vi "Lab Panel V5.10.vi"() -> ()   [LabVIEW 2013] (continued)
                          tunnel: w3985 -> [_ w4027]
                          tunnel: w3984 -> [_ w4019]
                          frame False {
                          }
                          frame True {
                            n2197 = local read "TDMS LAB02-1"() -> (w4032:refnum<k34>)
                            n2198 = Build Array(w4029) -> (w4024:dbl[])
                            n2199 = Build Array(w4027) -> (w4023:dbl[])
                            n2200 = Build Array(w4034) -> (w4022:dbl[])
                            n2201 = Build Array(w4035) -> (w4021:dbl[])
                            n2202 = Build Array(w4030) -> (w4026:dbl[])
                            n2203 = Build Array(w4028) -> (w4025:dbl[])
                            n2204 = Build Array(w4033) -> (w4020:dbl[])
                            n2205 = Build Array("AMPS ON", "AMPS OFF", "VOLTS", "PF", "TEMP Live", "TEMP Neut", "CYCLE") -> (w4003:string[])
                            n2206 = Bundle By Name("Y"=w4026, "t0"=w4019) -> (w4018:waveform(dbl))  [unwired: 1 in]
                            n2207 = Bundle By Name("Y"=w4025, "t0"=w4019) -> (w4017:waveform(dbl))  [unwired: 1 in]
                            n2208 = Bundle By Name("Y"=w4024, "t0"=w4019) -> (w4016:waveform(dbl))  [unwired: 1 in]
                            n2209 = Bundle By Name("Y"=w4023, "t0"=w4019) -> (w4015:waveform(dbl))  [unwired: 1 in]
                            n2210 = Bundle By Name("Y"=w4022, "t0"=w4019) -> (w4014:waveform(dbl))  [unwired: 1 in]
                            n2211 = Bundle By Name("Y"=w4021, "t0"=w4019) -> (w4013:waveform(dbl))  [unwired: 1 in]
                            n2212 = Bundle By Name("Y"=w4020, "t0"=w4019) -> (w4012:waveform(dbl))  [unwired: 1 in]
                            n2213 = Build Array(w4018, w4017, w4016, w4015, w4014, w4013, w4012) -> (w4011:waveform(dbl)[])
                            n2214 = TDMS Write(0:w4032, 5:"TEST VALUES", 7:w4003, 9:w4011) -> (4:w4002:refnum<k34>, 6:w4001:string, 15:w4000:errorcluster)  [unwired: 2 in, 1 out]
                            n2215 = TDMS Write(0:w4002, 5:w4001, 7:"TIME", 9:w3998, 11:w4000) -> (15:w3997:errorcluster)  [unwired: 1 in, 3 out]
                            n2216 = local write "data file error"(w3997) -> ()
                          }
                        }
                      }
                    }
                  }
                }
              }
              frame #3 {
                n2217 = case shown="True" w4036 {
                  tunnel: w4040 -> [_ w4045]
                  tunnel: w4039 -> [_ w4044]
                  tunnel: w4038 -> [_ w4042]
                  tunnel: w4037 -> [_ w4041]
                  frame False {
                  }
                  frame True {
                    n2218 = local read "DISP LAB02-2"() -> (w4046:T4)
                    n2219 = local read "SIG LAB02-2"() -> (w4047:T2)
                    n2220 = local read "ON L02-2"() -> (w4043:cluster{"amps":dbl, "volts":dbl, "pf":dbl})
                    n2221 = Unbundle(w4047) -> ("AMPS"=w4053:dbl, "VOLTS"=w4051:dbl, "PF"=w4050:dbl, "Tmp Live"=w4049:dbl, "Tmp Neut"=w4052:dbl)
                    n2222 = Unbundle(w4046) -> ("CYCLE"=w4048:dbl)  [unwired: 2 out]
                    n2223 = stacked-sequence {
                      tunnel: w4053 -> [w4057 w4076]
                      tunnel: w4052 -> [_ w4075]
                      tunnel: w4051 -> [w4056 w4074]
                      tunnel: w4050 -> [w4055 w4073]
                      tunnel: w4049 -> [_ w4072]
                      tunnel: w4048 -> [_ w4071]
                      tunnel: w4045 -> [_ w4070]
                      tunnel: w4044 -> [w4058 _]
                      tunnel: w4043 -> [w4054 w4068]
                      tunnel: w4042 -> [_ w4069]
                      tunnel: w4041 -> [_ w4064]
                      frame #0 {
                        n2224 = case shown="True" w4058 {
                          tunnel: w4057 -> [_ w4063]
                          tunnel: w4056 -> [_ w4062]
                          tunnel: w4055 -> [_ w4061]
                          tunnel: w4054 -> [_ w4059]
                          frame False {
                          }
                          frame True {
                            n2225 = Bundle(cluster=w4059, "amps"=w4063, "volts"=w4062, "pf"=w4061) -> (w4060:cluster{"amps":dbl, "volts":dbl, "pf":dbl})
                            n2226 = local write "ON L02-2"(w4060) -> ()
                          }
                        }
                      }
                      frame #1 {
                        n2227 = Unbundle(w4068) -> ("amps"=w4067:dbl, "volts"=w4066:dbl, "pf"=w4065:dbl)
                        n2228 = case shown="True" w4069 {
                          tunnel: w4076 -> [_ w4108]
                          tunnel: w4075 -> [_ w4115]
                          tunnel: w4074 -> [_ _]
                          tunnel: w4073 -> [_ _]
                          tunnel: w4072 -> [_ w4114]
                          tunnel: w4071 -> [_ w4113]
                          tunnel: w4070 -> [_ w4078]
                          tunnel: w4067 -> [_ w4110]
                          tunnel: w4066 -> [_ w4109]
                          tunnel: w4065 -> [_ w4107]
                          tunnel: w4064 -> [_ w4099]
                          frame False {
                          }
                          frame True {
                            n2229 = local read "TDMS LAB02-2"() -> (w4112:refnum<k34>)
                            n2230 = Build Array(w4109) -> (w4104:dbl[])
                            n2231 = Build Array(w4107) -> (w4103:dbl[])
                            n2232 = Build Array(w4114) -> (w4102:dbl[])
                            n2233 = Build Array(w4115) -> (w4101:dbl[])
                            n2234 = Build Array(w4110) -> (w4106:dbl[])
                            n2235 = Build Array(w4108) -> (w4105:dbl[])
                            n2236 = Build Array(w4113) -> (w4100:dbl[])
                            n2237 = Build Array("AMPS ON", "AMPS OFF", "VOLTS", "PF", "TEMP Live", "TEMP Neut", "CYCLE") -> (w4083:string[])
                            n2238 = Bundle By Name("Y"=w4106, "t0"=w4099) -> (w4098:waveform(dbl))  [unwired: 1 in]
                            n2239 = Bundle By Name("Y"=w4105, "t0"=w4099) -> (w4097:waveform(dbl))  [unwired: 1 in]
                            n2240 = Bundle By Name("Y"=w4104, "t0"=w4099) -> (w4096:waveform(dbl))  [unwired: 1 in]
                            n2241 = Bundle By Name("Y"=w4103, "t0"=w4099) -> (w4095:waveform(dbl))  [unwired: 1 in]
                            n2242 = Bundle By Name("Y"=w4102, "t0"=w4099) -> (w4094:waveform(dbl))  [unwired: 1 in]
                            n2243 = Bundle By Name("Y"=w4101, "t0"=w4099) -> (w4093:waveform(dbl))  [unwired: 1 in]
                            n2244 = Bundle By Name("Y"=w4100, "t0"=w4099) -> (w4092:waveform(dbl))  [unwired: 1 in]
                            n2245 = Build Array(w4098, w4097, w4096, w4095, w4094, w4093, w4092) -> (w4091:waveform(dbl)[])
                            n2246 = TDMS Write(0:w4112, 5:"TEST VALUES", 7:w4083, 9:w4091) -> (4:w4082:refnum<k34>, 6:w4081:string, 15:w4080:errorcluster)  [unwired: 2 in, 1 out]
                            n2247 = TDMS Write(0:w4082, 5:w4081, 7:"TIME", 9:w4078, 11:w4080) -> (15:w4077:errorcluster)  [unwired: 1 in, 3 out]
                            n2248 = local write "data file error"(w4077) -> ()
                          }
                        }
                      }
                    }
                  }
                }
              }
              frame #4 {
                n2249 = case shown="True" w4116 {
                  tunnel: w4120 -> [_ w4125]
                  tunnel: w4119 -> [_ w4124]
                  tunnel: w4118 -> [_ w4122]
                  tunnel: w4117 -> [_ w4121]
                  frame False {
                  }
                  frame True {
                    n2250 = local read "DISP LAB03-1"() -> (w4126:T4)
                    n2251 = local read "SIG LAB03-1"() -> (w4127:T2)
                    n2252 = local read "ON L03-1"() -> (w4123:cluster{"amps":dbl, "volts":dbl, "pf":dbl})
                    n2253 = Unbundle(w4127) -> ("AMPS"=w4133:dbl, "VOLTS"=w4131:dbl, "PF"=w4130:dbl, "Tmp Live"=w4129:dbl, "Tmp Neut"=w4132:dbl)
                    n2254 = Unbundle(w4126) -> ("CYCLE"=w4128:dbl)  [unwired: 2 out]
                    n2255 = stacked-sequence {
                      tunnel: w4133 -> [w4137 w4156]
                      tunnel: w4132 -> [_ w4155]
                      tunnel: w4131 -> [w4136 w4154]
                      tunnel: w4130 -> [w4135 w4153]
                      tunnel: w4129 -> [_ w4152]
                      tunnel: w4128 -> [_ w4151]
                      tunnel: w4125 -> [_ w4150]
                      tunnel: w4124 -> [w4138 _]
                      tunnel: w4123 -> [w4134 w4148]
                      tunnel: w4122 -> [_ w4149]
                      tunnel: w4121 -> [_ w4144]
                      frame #0 {
                        n2256 = case shown="True" w4138 {
                          tunnel: w4137 -> [_ w4143]
                          tunnel: w4136 -> [_ w4142]
                          tunnel: w4135 -> [_ w4141]
                          tunnel: w4134 -> [_ w4139]
                          frame False {
                          }
                          frame True {
                            n2257 = Bundle(cluster=w4139, "amps"=w4143, "volts"=w4142, "pf"=w4141) -> (w4140:cluster{"amps":dbl, "volts":dbl, "pf":dbl})
                            n2258 = local write "ON L03-1"(w4140) -> ()
                          }
                        }
                      }
                      frame #1 {
                        n2259 = Unbundle(w4148) -> ("amps"=w4147:dbl, "volts"=w4146:dbl, "pf"=w4145:dbl)
                        n2260 = case shown="True" w4149 {
                          tunnel: w4156 -> [_ w4188]
                          tunnel: w4155 -> [_ w4195]
                          tunnel: w4154 -> [_ _]
                          tunnel: w4153 -> [_ _]
                          tunnel: w4152 -> [_ w4194]
                          tunnel: w4151 -> [_ w4193]
                          tunnel: w4150 -> [_ w4158]
                          tunnel: w4147 -> [_ w4190]
                          tunnel: w4146 -> [_ w4189]
                          tunnel: w4145 -> [_ w4187]
                          tunnel: w4144 -> [_ w4179]
                          frame False {
                          }
                          frame True {
                            n2261 = local read "TDMS LAB03-1"() -> (w4192:refnum<k34>)
                            n2262 = Build Array(w4189) -> (w4184:dbl[])
                            n2263 = Build Array(w4187) -> (w4183:dbl[])
                            n2264 = Build Array(w4194) -> (w4182:dbl[])
                            n2265 = Build Array(w4195) -> (w4181:dbl[])
                            n2266 = Build Array(w4190) -> (w4186:dbl[])
                            n2267 = Build Array(w4188) -> (w4185:dbl[])
                            n2268 = Build Array(w4193) -> (w4180:dbl[])
                            n2269 = Build Array("AMPS ON", "AMPS OFF", "VOLTS", "PF", "TEMP Live", "TEMP Neut", "CYCLE") -> (w4163:string[])
                            n2270 = Bundle By Name("Y"=w4186, "t0"=w4179) -> (w4178:waveform(dbl))  [unwired: 1 in]
                            n2271 = Bundle By Name("Y"=w4185, "t0"=w4179) -> (w4177:waveform(dbl))  [unwired: 1 in]
                            n2272 = Bundle By Name("Y"=w4184, "t0"=w4179) -> (w4176:waveform(dbl))  [unwired: 1 in]
                            n2273 = Bundle By Name("Y"=w4183, "t0"=w4179) -> (w4175:waveform(dbl))  [unwired: 1 in]
                            n2274 = Bundle By Name("Y"=w4182, "t0"=w4179) -> (w4174:waveform(dbl))  [unwired: 1 in]
                            n2275 = Bundle By Name("Y"=w4181, "t0"=w4179) -> (w4173:waveform(dbl))  [unwired: 1 in]
                            n2276 = Bundle By Name("Y"=w4180, "t0"=w4179) -> (w4172:waveform(dbl))  [unwired: 1 in]
                            n2277 = Build Array(w4178, w4177, w4176, w4175, w4174, w4173, w4172) -> (w4171:waveform(dbl)[])
                            n2278 = TDMS Write(0:w4192, 5:"TEST VALUES", 7:w4163, 9:w4171) -> (4:w4162:refnum<k34>, 6:w4161:string, 15:w4160:errorcluster)  [unwired: 2 in, 1 out]
                            n2279 = TDMS Write(0:w4162, 5:w4161, 7:"TIME", 9:w4158, 11:w4160) -> (15:w4157:errorcluster)  [unwired: 1 in, 3 out]
                            n2280 = local write "data file error"(w4157) -> ()
                          }
                        }
                      }
                    }
                  }
                }
              }
              frame #5 {
                n2281 = case shown="True" w4196 {
                  tunnel: w4200 -> [_ w4205]
                  tunnel: w4199 -> [_ w4204]
                  tunnel: w4198 -> [_ w4202]
                  tunnel: w4197 -> [_ w4201]
                  frame False {
                  }
                  frame True {
                    n2282 = local read "DISP LAB03-2"() -> (w4206:T4)
                    n2283 = local read "SIG LAB03-2"() -> (w4207:T2)
                    n2284 = local read "ON L03-2"() -> (w4203:cluster{"amps":dbl, "volts":dbl, "pf":dbl})
                    n2285 = Unbundle(w4207) -> ("AMPS"=w4213:dbl, "VOLTS"=w4211:dbl, "PF"=w4210:dbl, "Tmp Live"=w4209:dbl, "Tmp Neut"=w4212:dbl)
                    n2286 = Unbundle(w4206) -> ("CYCLE"=w4208:dbl)  [unwired: 2 out]
                    n2287 = stacked-sequence {
                      tunnel: w4213 -> [w4217 w4236]
                      tunnel: w4212 -> [_ w4235]
                      tunnel: w4211 -> [w4216 w4234]
                      tunnel: w4210 -> [w4215 w4233]
                      tunnel: w4209 -> [_ w4232]
                      tunnel: w4208 -> [_ w4231]
                      tunnel: w4205 -> [_ w4230]
                      tunnel: w4204 -> [w4218 _]
                      tunnel: w4203 -> [w4214 w4228]
                      tunnel: w4202 -> [_ w4229]
                      tunnel: w4201 -> [_ w4224]
                      frame #0 {
                        n2288 = case shown="True" w4218 {
                          tunnel: w4217 -> [_ w4223]
                          tunnel: w4216 -> [_ w4222]
                          tunnel: w4215 -> [_ w4221]
                          tunnel: w4214 -> [_ w4219]
                          frame False {
                          }
                          frame True {
                            n2289 = Bundle(cluster=w4219, "amps"=w4223, "volts"=w4222, "pf"=w4221) -> (w4220:cluster{"amps":dbl, "volts":dbl, "pf":dbl})
                            n2290 = local write "ON L03-2"(w4220) -> ()
                          }
                        }
                      }
                      frame #1 {
                        n2291 = Unbundle(w4228) -> ("amps"=w4227:dbl, "volts"=w4226:dbl, "pf"=w4225:dbl)
                        n2292 = case shown="True" w4229 {
                          tunnel: w4236 -> [_ w4268]
                          tunnel: w4235 -> [_ w4275]
                          tunnel: w4234 -> [_ _]
                          tunnel: w4233 -> [_ _]
                          tunnel: w4232 -> [_ w4274]
                          tunnel: w4231 -> [_ w4273]
                          tunnel: w4230 -> [_ w4238]
                          tunnel: w4227 -> [_ w4270]
                          tunnel: w4226 -> [_ w4269]
                          tunnel: w4225 -> [_ w4267]
                          tunnel: w4224 -> [_ w4259]
                          frame False {
                          }
                          frame True {
                            n2293 = local read "TDMS LAB03-2"() -> (w4272:refnum<k34>)
                            n2294 = Build Array(w4269) -> (w4264:dbl[])
                            n2295 = Build Array(w4267) -> (w4263:dbl[])
                            n2296 = Build Array(w4274) -> (w4262:dbl[])
                            n2297 = Build Array(w4275) -> (w4261:dbl[])
                            n2298 = Build Array(w4270) -> (w4266:dbl[])
                            n2299 = Build Array(w4268) -> (w4265:dbl[])
                            n2300 = Build Array(w4273) -> (w4260:dbl[])
                            n2301 = Build Array("AMPS ON", "AMPS OFF", "VOLTS", "PF", "TEMP Live", "TEMP Neut", "CYCLE") -> (w4243:string[])
                            n2302 = Bundle By Name("Y"=w4266, "t0"=w4259) -> (w4258:waveform(dbl))  [unwired: 1 in]
                            n2303 = Bundle By Name("Y"=w4265, "t0"=w4259) -> (w4257:waveform(dbl))  [unwired: 1 in]
                            n2304 = Bundle By Name("Y"=w4264, "t0"=w4259) -> (w4256:waveform(dbl))  [unwired: 1 in]
                            n2305 = Bundle By Name("Y"=w4263, "t0"=w4259) -> (w4255:waveform(dbl))  [unwired: 1 in]
                            n2306 = Bundle By Name("Y"=w4262, "t0"=w4259) -> (w4254:waveform(dbl))  [unwired: 1 in]
                            n2307 = Bundle By Name("Y"=w4261, "t0"=w4259) -> (w4253:waveform(dbl))  [unwired: 1 in]
                            n2308 = Bundle By Name("Y"=w4260, "t0"=w4259) -> (w4252:waveform(dbl))  [unwired: 1 in]
                            n2309 = Build Array(w4258, w4257, w4256, w4255, w4254, w4253, w4252) -> (w4251:waveform(dbl)[])
                            n2310 = TDMS Write(0:w4272, 5:"TEST VALUES", 7:w4243, 9:w4251) -> (4:w4242:refnum<k34>, 6:w4241:string, 15:w4240:errorcluster)  [unwired: 2 in, 1 out]
                            n2311 = TDMS Write(0:w4242, 5:w4241, 7:"TIME", 9:w4238, 11:w4240) -> (15:w4237:errorcluster)  [unwired: 1 in, 3 out]
                            n2312 = local write "data file error"(w4237) -> ()
                          }
                        }
                      }
                    }
                  }
                }
              }
              frame #6 {
                n2313 = case shown="True" w4276 {
                  tunnel: w4280 -> [_ w4285]
                  tunnel: w4279 -> [_ w4284]
                  tunnel: w4278 -> [_ w4282]
                  tunnel: w4277 -> [_ w4281]
                  frame False {
                  }
                  frame True {
                    n2314 = local read "DISP LAB04-1"() -> (w4286:T4)
                    n2315 = local read "SIG LAB04-1"() -> (w4287:T2)
                    n2316 = local read "ON L04-1"() -> (w4283:cluster{"amps":dbl, "volts":dbl, "pf":dbl})
                    n2317 = Unbundle(w4287) -> ("AMPS"=w4293:dbl, "VOLTS"=w4291:dbl, "PF"=w4290:dbl, "Tmp Live"=w4289:dbl, "Tmp Neut"=w4292:dbl)
                    n2318 = Unbundle(w4286) -> ("CYCLE"=w4288:dbl)  [unwired: 2 out]
                    n2319 = stacked-sequence {
                      tunnel: w4293 -> [w4297 w4316]
                      tunnel: w4292 -> [_ w4315]
                      tunnel: w4291 -> [w4296 w4314]
                      tunnel: w4290 -> [w4295 w4313]
                      tunnel: w4289 -> [_ w4312]
                      tunnel: w4288 -> [_ w4311]
                      tunnel: w4285 -> [_ w4310]
                      tunnel: w4284 -> [w4298 _]
                      tunnel: w4283 -> [w4294 w4308]
                      tunnel: w4282 -> [_ w4309]
                      tunnel: w4281 -> [_ w4304]
                      frame #0 {
                        n2320 = case shown="True" w4298 {
                          tunnel: w4297 -> [_ w4303]
                          tunnel: w4296 -> [_ w4302]
                          tunnel: w4295 -> [_ w4301]
                          tunnel: w4294 -> [_ w4299]
                          frame False {
                          }
                          frame True {
                            n2321 = Bundle(cluster=w4299, "amps"=w4303, "volts"=w4302, "pf"=w4301) -> (w4300:cluster{"amps":dbl, "volts":dbl, "pf":dbl})
                            n2322 = local write "ON L04-1"(w4300) -> ()
                          }
                        }
                      }
                      frame #1 {
                        n2323 = Unbundle(w4308) -> ("amps"=w4307:dbl, "volts"=w4306:dbl, "pf"=w4305:dbl)
                        n2324 = case shown="True" w4309 {
                          tunnel: w4316 -> [_ w4348]
                          tunnel: w4315 -> [_ w4355]
                          tunnel: w4314 -> [_ _]
                          tunnel: w4313 -> [_ _]
                          tunnel: w4312 -> [_ w4354]
                          tunnel: w4311 -> [_ w4353]
                          tunnel: w4310 -> [_ w4318]
                          tunnel: w4307 -> [_ w4350]
                          tunnel: w4306 -> [_ w4349]
                          tunnel: w4305 -> [_ w4347]
                          tunnel: w4304 -> [_ w4339]
                          frame False {
                          }
                          frame True {
                            n2325 = local read "TDMS LAB04-1"() -> (w4352:refnum<k34>)
                            n2326 = Build Array(w4349) -> (w4344:dbl[])
                            n2327 = Build Array(w4347) -> (w4343:dbl[])
                            n2328 = Build Array(w4354) -> (w4342:dbl[])
                            n2329 = Build Array(w4355) -> (w4341:dbl[])
                            n2330 = Build Array(w4350) -> (w4346:dbl[])
                            n2331 = Build Array(w4348) -> (w4345:dbl[])
                            n2332 = Build Array(w4353) -> (w4340:dbl[])
                            n2333 = Build Array("AMPS ON", "AMPS OFF", "VOLTS", "PF", "TEMP Live", "TEMP Neut", "CYCLE") -> (w4323:string[])
                            n2334 = Bundle By Name("Y"=w4346, "t0"=w4339) -> (w4338:waveform(dbl))  [unwired: 1 in]
                            n2335 = Bundle By Name("Y"=w4345, "t0"=w4339) -> (w4337:waveform(dbl))  [unwired: 1 in]
                            n2336 = Bundle By Name("Y"=w4344, "t0"=w4339) -> (w4336:waveform(dbl))  [unwired: 1 in]
                            n2337 = Bundle By Name("Y"=w4343, "t0"=w4339) -> (w4335:waveform(dbl))  [unwired: 1 in]
                            n2338 = Bundle By Name("Y"=w4342, "t0"=w4339) -> (w4334:waveform(dbl))  [unwired: 1 in]
                            n2339 = Bundle By Name("Y"=w4341, "t0"=w4339) -> (w4333:waveform(dbl))  [unwired: 1 in]
                            n2340 = Bundle By Name("Y"=w4340, "t0"=w4339) -> (w4332:waveform(dbl))  [unwired: 1 in]
                            n2341 = Build Array(w4338, w4337, w4336, w4335, w4334, w4333, w4332) -> (w4331:waveform(dbl)[])
                            n2342 = TDMS Write(0:w4352, 5:"TEST VALUES", 7:w4323, 9:w4331) -> (4:w4322:refnum<k34>, 6:w4321:string, 15:w4320:errorcluster)  [unwired: 2 in, 1 out]
                            n2343 = TDMS Write(0:w4322, 5:w4321, 7:"TIME", 9:w4318, 11:w4320) -> (15:w4317:errorcluster)  [unwired: 1 in, 3 out]
                            n2344 = local write "data file error"(w4317) -> ()
                          }
                        }
                      }
                    }
                  }
                }
              }
              frame #7 {
                n2345 = case shown="True" w4356 {
                  tunnel: w4360 -> [_ w4365]
                  tunnel: w4359 -> [_ w4364]
                  tunnel: w4358 -> [_ w4362]
                  tunnel: w4357 -> [_ w4361]
                  frame False {
                  }
                  frame True {
                    n2346 = local read "DISP LAB04-2"() -> (w4366:T4)
                    n2347 = local read "SIG LAB04-2"() -> (w4367:T2)
                    n2348 = local read "ON L04-2"() -> (w4363:cluster{"amps":dbl, "volts":dbl, "pf":dbl})
                    n2349 = Unbundle(w4367) -> ("AMPS"=w4373:dbl, "VOLTS"=w4371:dbl, "PF"=w4370:dbl, "Tmp Live"=w4369:dbl, "Tmp Neut"=w4372:dbl)
                    n2350 = Unbundle(w4366) -> ("CYCLE"=w4368:dbl)  [unwired: 2 out]
                    n2351 = stacked-sequence {
                      tunnel: w4373 -> [w4377 w4396]
                      tunnel: w4372 -> [_ w4395]
                      tunnel: w4371 -> [w4376 w4394]
                      tunnel: w4370 -> [w4375 w4393]
                      tunnel: w4369 -> [_ w4392]
                      tunnel: w4368 -> [_ w4391]
                      tunnel: w4365 -> [_ w4390]
                      tunnel: w4364 -> [w4378 _]
                      tunnel: w4363 -> [w4374 w4388]
                      tunnel: w4362 -> [_ w4389]
                      tunnel: w4361 -> [_ w4384]
                      frame #0 {
                        n2352 = case shown="True" w4378 {
                          tunnel: w4377 -> [_ w4383]
                          tunnel: w4376 -> [_ w4382]
                          tunnel: w4375 -> [_ w4381]
                          tunnel: w4374 -> [_ w4379]
                          frame False {
                          }
                          frame True {
                            n2353 = Bundle(cluster=w4379, "amps"=w4383, "volts"=w4382, "pf"=w4381) -> (w4380:cluster{"amps":dbl, "volts":dbl, "pf":dbl})
                            n2354 = local write "ON L04-2"(w4380) -> ()
                          }
                        }
                      }
                      frame #1 {
                        n2355 = Unbundle(w4388) -> ("amps"=w4387:dbl, "volts"=w4386:dbl, "pf"=w4385:dbl)
                        n2356 = case shown="True" w4389 {
                          tunnel: w4396 -> [_ w4428]
                          tunnel: w4395 -> [_ w4435]
                          tunnel: w4394 -> [_ _]
                          tunnel: w4393 -> [_ _]
                          tunnel: w4392 -> [_ w4434]
                          tunnel: w4391 -> [_ w4433]
                          tunnel: w4390 -> [_ w4398]
                          tunnel: w4387 -> [_ w4430]
                          tunnel: w4386 -> [_ w4429]
                          tunnel: w4385 -> [_ w4427]
                          tunnel: w4384 -> [_ w4419]
                          frame False {
                          }
                          frame True {
                            n2357 = local read "TDMS LAB04-2"() -> (w4432:refnum<k34>)
                            n2358 = Build Array(w4429) -> (w4424:dbl[])
                            n2359 = Build Array(w4427) -> (w4423:dbl[])
                            n2360 = Build Array(w4434) -> (w4422:dbl[])
                            n2361 = Build Array(w4435) -> (w4421:dbl[])
                            n2362 = Build Array(w4430) -> (w4426:dbl[])
                            n2363 = Build Array(w4428) -> (w4425:dbl[])
                            n2364 = Build Array(w4433) -> (w4420:dbl[])
                            n2365 = Build Array("AMPS ON", "AMPS OFF", "VOLTS", "PF", "TEMP Live", "TEMP Neut", "CYCLE") -> (w4403:string[])
                            n2366 = Bundle By Name("Y"=w4426, "t0"=w4419) -> (w4418:waveform(dbl))  [unwired: 1 in]
                            n2367 = Bundle By Name("Y"=w4425, "t0"=w4419) -> (w4417:waveform(dbl))  [unwired: 1 in]
                            n2368 = Bundle By Name("Y"=w4424, "t0"=w4419) -> (w4416:waveform(dbl))  [unwired: 1 in]
                            n2369 = Bundle By Name("Y"=w4423, "t0"=w4419) -> (w4415:waveform(dbl))  [unwired: 1 in]
                            n2370 = Bundle By Name("Y"=w4422, "t0"=w4419) -> (w4414:waveform(dbl))  [unwired: 1 in]
                            n2371 = Bundle By Name("Y"=w4421, "t0"=w4419) -> (w4413:waveform(dbl))  [unwired: 1 in]
                            n2372 = Bundle By Name("Y"=w4420, "t0"=w4419) -> (w4412:waveform(dbl))  [unwired: 1 in]
                            n2373 = Build Array(w4418, w4417, w4416, w4415, w4414, w4413, w4412) -> (w4411:waveform(dbl)[])
                            n2374 = TDMS Write(0:w4432, 5:"TEST VALUES", 7:w4403, 9:w4411) -> (4:w4402:refnum<k34>, 6:w4401:string, 15:w4400:errorcluster)  [unwired: 2 in, 1 out]
                            n2375 = TDMS Write(0:w4402, 5:w4401, 7:"TIME", 9:w4398, 11:w4400) -> (15:w4397:errorcluster)  [unwired: 1 in, 3 out]
                            n2376 = local write "data file error"(w4397) -> ()
                          }
                        }
                      }
                    }
                  }
                }
              }
              frame #8 {
                n2377 = case shown="True" w4436 {
                  tunnel: w4440 -> [_ w4445]
                  tunnel: w4439 -> [_ w4444]
                  tunnel: w4438 -> [_ w4442]
                  tunnel: w4437 -> [_ w4441]
                  frame False {
                  }
                  frame True {
                    n2378 = local read "DISP LAB05-1"() -> (w4446:T4)
                    n2379 = local read "SIG LAB05-1"() -> (w4447:T2)
                    n2380 = local read "ON L05-1"() -> (w4443:cluster{"amps":dbl, "volts":dbl, "pf":dbl})
                    n2381 = Unbundle(w4447) -> ("AMPS"=w4453:dbl, "VOLTS"=w4451:dbl, "PF"=w4450:dbl, "Tmp Live"=w4449:dbl, "Tmp Neut"=w4452:dbl)
                    n2382 = Unbundle(w4446) -> ("CYCLE"=w4448:dbl)  [unwired: 2 out]
                    n2383 = stacked-sequence {
                      tunnel: w4453 -> [w4457 w4476]
                      tunnel: w4452 -> [_ w4475]
                      tunnel: w4451 -> [w4456 w4474]
                      tunnel: w4450 -> [w4455 w4473]
                      tunnel: w4449 -> [_ w4472]
                      tunnel: w4448 -> [_ w4471]
                      tunnel: w4445 -> [_ w4470]
                      tunnel: w4444 -> [w4458 _]
                      tunnel: w4443 -> [w4454 w4468]
                      tunnel: w4442 -> [_ w4469]
                      tunnel: w4441 -> [_ w4464]
                      frame #0 {
                        n2384 = case shown="True" w4458 {
                          tunnel: w4457 -> [_ w4463]
                          tunnel: w4456 -> [_ w4462]
                          tunnel: w4455 -> [_ w4461]
                          tunnel: w4454 -> [_ w4459]
                          frame False {
                          }
                          frame True {
                            n2385 = Bundle(cluster=w4459, "amps"=w4463, "volts"=w4462, "pf"=w4461) -> (w4460:cluster{"amps":dbl, "volts":dbl, "pf":dbl})
                            n2386 = local write "ON L05-1"(w4460) -> ()
                          }
                        }
                      }
                      frame #1 {
                        n2387 = Unbundle(w4468) -> ("amps"=w4467:dbl, "volts"=w4466:dbl, "pf"=w4465:dbl)
                        n2388 = case shown="True" w4469 {
                          tunnel: w4476 -> [_ w4508]
                          tunnel: w4475 -> [_ w4515]
                          tunnel: w4474 -> [_ _]
                          tunnel: w4473 -> [_ _]
                          tunnel: w4472 -> [_ w4514]
                          tunnel: w4471 -> [_ w4513]
                          tunnel: w4470 -> [_ w4478]
                          tunnel: w4467 -> [_ w4510]
                          tunnel: w4466 -> [_ w4509]
                          tunnel: w4465 -> [_ w4507]
                          tunnel: w4464 -> [_ w4499]
                          frame False {
                          }
                          frame True {
                            n2389 = local read "TDMS LAB05-1"() -> (w4512:refnum<k34>)
                            n2390 = Build Array(w4509) -> (w4504:dbl[])
                            n2391 = Build Array(w4507) -> (w4503:dbl[])
                            n2392 = Build Array(w4514) -> (w4502:dbl[])
                            n2393 = Build Array(w4515) -> (w4501:dbl[])
                            n2394 = Build Array(w4510) -> (w4506:dbl[])
                            n2395 = Build Array(w4508) -> (w4505:dbl[])
                            n2396 = Build Array(w4513) -> (w4500:dbl[])
                            n2397 = Build Array("AMPS ON", "AMPS OFF", "VOLTS", "PF", "TEMP Live", "TEMP Neut", "CYCLE") -> (w4483:string[])
                            n2398 = Bundle By Name("Y"=w4506, "t0"=w4499) -> (w4498:waveform(dbl))  [unwired: 1 in]
                            n2399 = Bundle By Name("Y"=w4505, "t0"=w4499) -> (w4497:waveform(dbl))  [unwired: 1 in]
                            n2400 = Bundle By Name("Y"=w4504, "t0"=w4499) -> (w4496:waveform(dbl))  [unwired: 1 in]
                            n2401 = Bundle By Name("Y"=w4503, "t0"=w4499) -> (w4495:waveform(dbl))  [unwired: 1 in]
                            n2402 = Bundle By Name("Y"=w4502, "t0"=w4499) -> (w4494:waveform(dbl))  [unwired: 1 in]
                            n2403 = Bundle By Name("Y"=w4501, "t0"=w4499) -> (w4493:waveform(dbl))  [unwired: 1 in]
                            n2404 = Bundle By Name("Y"=w4500, "t0"=w4499) -> (w4492:waveform(dbl))  [unwired: 1 in]
                            n2405 = Build Array(w4498, w4497, w4496, w4495, w4494, w4493, w4492) -> (w4491:waveform(dbl)[])
                            n2406 = TDMS Write(0:w4512, 5:"TEST VALUES", 7:w4483, 9:w4491) -> (4:w4482:refnum<k34>, 6:w4481:string, 15:w4480:errorcluster)  [unwired: 2 in, 1 out]
                            n2407 = TDMS Write(0:w4482, 5:w4481, 7:"TIME", 9:w4478, 11:w4480) -> (15:w4477:errorcluster)  [unwired: 1 in, 3 out]
                            n2408 = local write "data file error"(w4477) -> ()
                          }
                        }
                      }
                    }
                  }
                }
              }
              frame #9 {
                n2409 = case shown="True" w4516 {
                  tunnel: w4520 -> [_ w4525]
                  tunnel: w4519 -> [_ w4524]
                  tunnel: w4518 -> [_ w4522]
                  tunnel: w4517 -> [_ w4521]
                  frame False {
                  }
                  frame True {
                    n2410 = local read "DISP LAB05-2"() -> (w4526:T4)
                    n2411 = local read "SIG LAB05-2"() -> (w4527:T2)
                    n2412 = local read "ON L05-2"() -> (w4523:cluster{"amps":dbl, "volts":dbl, "pf":dbl})
                    n2413 = Unbundle(w4527) -> ("AMPS"=w4533:dbl, "VOLTS"=w4531:dbl, "PF"=w4530:dbl, "Tmp Live"=w4529:dbl, "Tmp Neut"=w4532:dbl)
                    n2414 = Unbundle(w4526) -> ("CYCLE"=w4528:dbl)  [unwired: 2 out]
                    n2415 = stacked-sequence {
                      tunnel: w4533 -> [w4537 w4556]
                      tunnel: w4532 -> [_ w4555]
                      tunnel: w4531 -> [w4536 w4554]
                      tunnel: w4530 -> [w4535 w4553]
                      tunnel: w4529 -> [_ w4552]
                      tunnel: w4528 -> [_ w4551]
                      tunnel: w4525 -> [_ w4550]
                      tunnel: w4524 -> [w4538 _]
                      tunnel: w4523 -> [w4534 w4548]
                      tunnel: w4522 -> [_ w4549]
                      tunnel: w4521 -> [_ w4544]
                      frame #0 {
                        n2416 = case shown="True" w4538 {
                          tunnel: w4537 -> [_ w4543]
                          tunnel: w4536 -> [_ w4542]
                          tunnel: w4535 -> [_ w4541]
                          tunnel: w4534 -> [_ w4539]
                          frame False {
                          }
                          frame True {
                            n2417 = Bundle(cluster=w4539, "amps"=w4543, "volts"=w4542, "pf"=w4541) -> (w4540:cluster{"amps":dbl, "volts":dbl, "pf":dbl})
                            n2418 = local write "ON L05-2"(w4540) -> ()
                          }
                        }
                      }
                      frame #1 {
                        n2419 = Unbundle(w4548) -> ("amps"=w4547:dbl, "volts"=w4546:dbl, "pf"=w4545:dbl)
                        n2420 = case shown="True" w4549 {
                          tunnel: w4556 -> [_ w4588]
                          tunnel: w4555 -> [_ w4595]
                          tunnel: w4554 -> [_ _]
                          tunnel: w4553 -> [_ _]
                          tunnel: w4552 -> [_ w4594]
                          tunnel: w4551 -> [_ w4593]
                          tunnel: w4550 -> [_ w4558]
                          tunnel: w4547 -> [_ w4590]
                          tunnel: w4546 -> [_ w4589]
                          tunnel: w4545 -> [_ w4587]
                          tunnel: w4544 -> [_ w4579]
                          frame False {
                          }
                          frame True {
                            n2421 = local read "TDMS LAB05-2"() -> (w4592:refnum<k34>)
                            n2422 = Build Array(w4589) -> (w4584:dbl[])
                            n2423 = Build Array(w4587) -> (w4583:dbl[])
                            n2424 = Build Array(w4594) -> (w4582:dbl[])
                            n2425 = Build Array(w4595) -> (w4581:dbl[])
                            n2426 = Build Array(w4590) -> (w4586:dbl[])
                            n2427 = Build Array(w4588) -> (w4585:dbl[])
                            n2428 = Build Array(w4593) -> (w4580:dbl[])
                            n2429 = Build Array("AMPS ON", "AMPS OFF", "VOLTS", "PF", "TEMP Live", "TEMP Neut", "CYCLE") -> (w4563:string[])
                            n2430 = Bundle By Name("Y"=w4586, "t0"=w4579) -> (w4578:waveform(dbl))  [unwired: 1 in]
                            n2431 = Bundle By Name("Y"=w4585, "t0"=w4579) -> (w4577:waveform(dbl))  [unwired: 1 in]
                            n2432 = Bundle By Name("Y"=w4584, "t0"=w4579) -> (w4576:waveform(dbl))  [unwired: 1 in]
                            n2433 = Bundle By Name("Y"=w4583, "t0"=w4579) -> (w4575:waveform(dbl))  [unwired: 1 in]
                            n2434 = Bundle By Name("Y"=w4582, "t0"=w4579) -> (w4574:waveform(dbl))  [unwired: 1 in]
                            n2435 = Bundle By Name("Y"=w4581, "t0"=w4579) -> (w4573:waveform(dbl))  [unwired: 1 in]
                            n2436 = Bundle By Name("Y"=w4580, "t0"=w4579) -> (w4572:waveform(dbl))  [unwired: 1 in]
                            n2437 = Build Array(w4578, w4577, w4576, w4575, w4574, w4573, w4572) -> (w4571:waveform(dbl)[])
                            n2438 = TDMS Write(0:w4592, 5:"TEST VALUES", 7:w4563, 9:w4571) -> (4:w4562:refnum<k34>, 6:w4561:string, 15:w4560:errorcluster)  [unwired: 2 in, 1 out]
                            n2439 = TDMS Write(0:w4562, 5:w4561, 7:"TIME", 9:w4558, 11:w4560) -> (15:w4557:errorcluster)  [unwired: 1 in, 3 out]
                            n2440 = local write "data file error"(w4557) -> ()
                          }
                        }
                      }
                    }
                  }
                }
              }
            }
          }
          frame #13 {
            # "display test values on chart"
            n2441 = local read "jig cycle"() -> (w4600:dbl)
            n2442 = local read "on loops"() -> (w4602:dbl)
            n2443 = Add(x=w4602, y=2) -> (x+y=w4599:dbl)
            n2444 = Equal?(x=w4600, y=1) -> (x = y?=w4598:bool)
            n2445 = Equal?(x=w4600, y=w4599) -> (x = y?=w4597:bool)
            n2446 = Or(x=w4598, y=w4597) -> (x .or. y?=w4596:bool)
            "graph flag" <- w4596
            n2447 = global write "Global display 3.vi" "graph flag"(w4596) -> ()
            n2448 = case shown="True" w4596 {
              frame False {
              }
              frame True {
                n2449 = local read "SIG LAB05-1"() -> (w4645:T2)
                n2450 = local read "SIG LAB04-2"() -> (w4646:T2)
                n2451 = local read "SIG LAB05-2"() -> (w4644:T2)
                n2452 = local read "SIG LAB04-1"() -> (w4647:T2)
                n2453 = local read "SIG LAB03-1"() -> (w4649:T2)
                n2454 = local read "SIG LAB03-2"() -> (w4648:T2)
                n2455 = local read "SIG LAB01-1"() -> (w4653:T2)
                n2456 = local read "SIG LAB02-2"() -> (w4650:T2)
                n2457 = local read "SIG LAB02-1"() -> (w4651:T2)
                n2458 = local read "SIG LAB01-2"() -> (w4652:T2)
                n2459 = Unbundle(w4646) -> ("AMPS"=w4636:dbl, "VOLTS"=w4626:dbl, "Tmp Live"=w4616:dbl, "Tmp Neut"=w4606:dbl)  [unwired: 1 out]
                n2460 = Unbundle(w4645) -> ("AMPS"=w4635:dbl, "VOLTS"=w4625:dbl, "Tmp Live"=w4615:dbl, "Tmp Neut"=w4605:dbl)  [unwired: 1 out]
                n2461 = Unbundle(w4644) -> ("AMPS"=w4634:dbl, "VOLTS"=w4624:dbl, "Tmp Live"=w4614:dbl, "Tmp Neut"=w4604:dbl)  [unwired: 1 out]
                n2462 = Unbundle(w4647) -> ("AMPS"=w4637:dbl, "VOLTS"=w4627:dbl, "Tmp Live"=w4617:dbl, "Tmp Neut"=w4607:dbl)  [unwired: 1 out]
                n2463 = Unbundle(w4648) -> ("AMPS"=w4638:dbl, "VOLTS"=w4628:dbl, "Tmp Live"=w4618:dbl, "Tmp Neut"=w4608:dbl)  [unwired: 1 out]
                n2464 = Unbundle(w4649) -> ("AMPS"=w4639:dbl, "VOLTS"=w4629:dbl, "Tmp Live"=w4619:dbl, "Tmp Neut"=w4609:dbl)  [unwired: 1 out]
                n2465 = Unbundle(w4650) -> ("AMPS"=w4640:dbl, "VOLTS"=w4630:dbl, "Tmp Live"=w4620:dbl, "Tmp Neut"=w4610:dbl)  [unwired: 1 out]
                n2466 = Unbundle(w4651) -> ("AMPS"=w4641:dbl, "VOLTS"=w4631:dbl, "Tmp Live"=w4621:dbl, "Tmp Neut"=w4611:dbl)  [unwired: 1 out]
                n2467 = Unbundle(w4653) -> ("AMPS"=w4643:dbl, "VOLTS"=w4633:dbl, "Tmp Live"=w4623:dbl, "Tmp Neut"=w4613:dbl)  [unwired: 1 out]
                n2468 = Unbundle(w4652) -> ("AMPS"=w4642:dbl, "VOLTS"=w4632:dbl, "Tmp Live"=w4622:dbl, "Tmp Neut"=w4612:dbl)  [unwired: 1 out]
                n2469 = stacked-sequence {
                  tunnel: w4643 -> [w4685 _ _]
                  tunnel: w4642 -> [w4684 _ _]
                  tunnel: w4641 -> [w4675 _ _]
                  tunnel: w4640 -> [w4674 _ _]
                  tunnel: w4639 -> [w4664 _ _]
                  tunnel: w4638 -> [w4663 _ _]
                  tunnel: w4637 -> [_ w4708 _]
                  tunnel: w4636 -> [_ w4707 _]
                  tunnel: w4635 -> [_ w4697 _]
                  tunnel: w4634 -> [_ w4696 _]
                  tunnel: w4633 -> [w4682 _ _]
                  tunnel: w4632 -> [w4681 _ _]
                  tunnel: w4631 -> [w4672 _ _]
                  tunnel: w4630 -> [w4671 _ _]
                  tunnel: w4629 -> [w4662 _ _]
                  tunnel: w4628 -> [w4661 _ _]
                  tunnel: w4627 -> [_ w4706 _]
                  tunnel: w4626 -> [_ w4705 _]
                  tunnel: w4625 -> [_ w4695 _]
                  tunnel: w4624 -> [_ w4694 _]
                  tunnel: w4623 -> [w4679 _ _]
                  tunnel: w4622 -> [w4677 _ _]
                  tunnel: w4621 -> [w4668 _ _]
                  tunnel: w4620 -> [w4666 _ _]
                  tunnel: w4619 -> [w4660 _ _]
                  tunnel: w4618 -> [w4658 _ _]
                  tunnel: w4617 -> [_ w4704 _]
                  tunnel: w4616 -> [_ w4702 _]
                  tunnel: w4615 -> [_ w4693 _]
                  tunnel: w4614 -> [_ w4691 _]
                  tunnel: w4613 -> [w4678 _ _]
                  tunnel: w4612 -> [w4676 _ _]
                  tunnel: w4611 -> [w4667 _ _]
                  tunnel: w4610 -> [w4665 _ _]
                  tunnel: w4609 -> [w4659 _ _]
                  tunnel: w4608 -> [w4657 _ _]
                  tunnel: w4607 -> [_ w4703 _]
                  tunnel: w4606 -> [_ w4701 _]
                  tunnel: w4605 -> [_ w4692 _]
                  tunnel: w4604 -> [_ w4690 _]
                  frame #0 {
                    n2470 = Merge Signals(w4685, w4684) -> (→"LAB01 AMPS":dynamicdata)
                    n2471 = Merge Signals(w4682, w4681) -> (→"LAB01 VOLTS":dynamicdata)
                    n2472 = Merge Signals(w4662, w4661) -> (→"LAB03 VOLTS":dynamicdata)
                    n2473 = Merge Signals(w4679, w4678, w4677, w4676) -> (→"LAB01 deg C":dynamicdata)
                    n2474 = Merge Signals(w4675, w4674) -> (→"LAB02 AMPS":dynamicdata)
                    n2475 = Merge Signals(w4668, w4667, w4666, w4665) -> (→"LAB02 deg C":dynamicdata)
                    n2476 = Merge Signals(w4660, w4659, w4658, w4657) -> (→"LAB03 deg C":dynamicdata)
                    n2477 = Merge Signals(w4672, w4671) -> (→"LAB02 VOLTS":dynamicdata)
                    n2478 = Merge Signals(w4664, w4663) -> (→"LAB03 AMPS":dynamicdata)
                  }
                  frame #1 {
                    n2479 = Merge Signals(w4695, w4694) -> (→"LAB05 VOLTS":dynamicdata)
                    n2480 = Merge Signals(w4708, w4707) -> (→"LAB04 AMPS":dynamicdata)
                    n2481 = Merge Signals(w4697, w4696) -> (→"LAB05 AMPS":dynamicdata)
                    n2482 = Merge Signals(w4693, w4692, w4691, w4690) -> (→"LAB05 deg C":dynamicdata)
                    n2483 = Merge Signals(w4704, w4703, w4702, w4701) -> (→"LAB04 deg C":dynamicdata)
                    n2484 = Merge Signals(w4706, w4705) -> (→"LAB04 VOLTS":dynamicdata)
                  }
                  frame #2 {
                    n2485 = local read "LAB05 VOLTS"() -> (w4716:dynamicdata)
                    n2486 = local read "LAB04 VOLTS"() -> (w4717:dynamicdata)
                    n2487 = local read "LAB02 VOLTS"() -> (w4719:dynamicdata)
                    n2488 = local read "LAB03 VOLTS"() -> (w4718:dynamicdata)
                    n2489 = local read "LAB05 AMPS"() -> (w4722:dynamicdata)
                    n2490 = local read "LAB01 VOLTS"() -> (w4720:dynamicdata)
                    n2491 = local read "LAB04 AMPS"() -> (w4723:dynamicdata)
                    n2492 = local read "LAB03 AMPS"() -> (w4724:dynamicdata)
                    n2493 = local read "LAB03 deg C"() -> (w4712:dynamicdata)
                    n2494 = local read "LAB02 AMPS"() -> (w4725:dynamicdata)
                    n2495 = local read "LAB04 deg C"() -> (w4711:dynamicdata)
                    n2496 = local read "LAB05 deg C"() -> (w4710:dynamicdata)
                    n2497 = local read "LAB02 deg C"() -> (w4713:dynamicdata)
                    n2498 = local read "LAB01 deg C"() -> (w4714:dynamicdata)
                    n2499 = local read "LAB01 AMPS"() -> (w4726:dynamicdata)
                    n2500 = Merge Signals(w4714, w4713, w4712, w4711, w4710) -> (w4709:dynamicdata)
                    n2501 = Merge Signals(w4726, w4725, w4724, w4723, w4722) -> (w4721:dynamicdata)
                    n2502 = Merge Signals(w4720, w4719, w4718, w4717, w4716) -> (w4715:dynamicdata)
                    n2503 = global write "Global display 3.vi" "graph volts"(w4715) -> ()
                    n2504 = global write "Global display 3.vi" "graph deg C"(w4709) -> ()
                    n2505 = global write "Global display 3.vi" "graph amps"(w4721) -> ()
                  }
                }
              }
            }
          }
          frame #14 {
            # "check for amps fail"
            # "check for cycle test & temperature rise fail conditions"
            n2506 = local read "on loops"() -> (w4753:dbl)
            n2507 = local read "jig cycle"() -> (w4750:dbl)
            n2508 = local read "jig cycle"() -> (w4755:dbl)
            n2509 = Add(x=w4753, y=3.0) -> (x+y=w4751:dbl)
            n2510 = Equal?(x=w4750, y=w4751) -> (x = y?=w4746:bool)
            n2511 = local read "Fail Loops"() -> (w4727:dbl)
            n2512 = Equal?(x=w4755, y=1.0) -> (x = y?=w4748:bool)
            n2513 = global write "Global 1.vi" "fail count"(w4727) -> ()
            n2514 = stacked-sequence {
              tunnel: w4749 -> [w4758 _ _ _ _ _ _ _ _ _]
              tunnel: w4748 -> [w4759 w4779 w4799 w4819 w4839 w4859 w4879 w4899 w4919 w4939]
              tunnel: w4747 -> [w4756 _ _ _ _ _ _ _ _ _]
              tunnel: w4746 -> [w4757 w4778 w4798 w4818 w4838 w4858 w4878 w4898 w4918 w4938]
              tunnel: w4745 -> [_ w4777 _ _ _ _ _ _ _ _]
              tunnel: w4744 -> [_ w4776 _ _ _ _ _ _ _ _]
              tunnel: w4743 -> [_ _ w4797 _ _ _ _ _ _ _]
              tunnel: w4742 -> [_ _ w4796 _ _ _ _ _ _ _]
              tunnel: w4741 -> [_ _ _ w4817 _ _ _ _ _ _]
              tunnel: w4740 -> [_ _ _ w4816 _ _ _ _ _ _]
              tunnel: w4739 -> [_ _ _ _ w4837 _ _ _ _ _]
              tunnel: w4738 -> [_ _ _ _ w4836 _ _ _ _ _]
              tunnel: w4737 -> [_ _ _ _ _ w4857 _ _ _ _]
              tunnel: w4736 -> [_ _ _ _ _ w4856 _ _ _ _]
              tunnel: w4735 -> [_ _ _ _ _ _ w4877 _ _ _]
              tunnel: w4734 -> [_ _ _ _ _ _ w4876 _ _ _]
              tunnel: w4733 -> [_ _ _ _ _ _ _ w4897 _ _]
              tunnel: w4732 -> [_ _ _ _ _ _ _ w4896 _ _]
              tunnel: w4731 -> [_ _ _ _ _ _ _ _ w4917 _]
              tunnel: w4730 -> [_ _ _ _ _ _ _ _ w4916 _]
              tunnel: w4729 -> [_ _ _ _ _ _ _ _ _ w4937]
              tunnel: w4728 -> [_ _ _ _ _ _ _ _ _ w4936]
              frame #0 {
                # "LAB01-1"
                n2515 = case shown="True" w4756 {
                  tunnel: w4759 -> [_ w4772]
                  tunnel: w4758 -> [_ w4769]
                  tunnel: w4757 -> [_ w4768]
                  frame False {
                  }
                  frame True {
                    n2516 = local read "TEMP START LAB01-1"() -> (w4774:cluster{"TL":dbl, "TN":dbl})
                    n2517 = local read "RESULT LAB01-1"() -> (w4763:bool)
                    n2518 = local read "FAIL LAB01-1"() -> (w4766:cluster{"LO":dbl, "HI":dbl})
                    n2519 = local read "TDMS LAB01-1"() -> (w4773:refnum<k34>)
